vi "Estimate Signal Amplitude and Offset - Sine.vi"(9 "number of bits":i32, 10 "ideal code width":dbl, 11 "histogram":i32[](array[numeric])) -> (2 "estimated offset":dbl, 3 "estimated amplitude (pk-pk)":dbl)   [LabVIEW 2021]
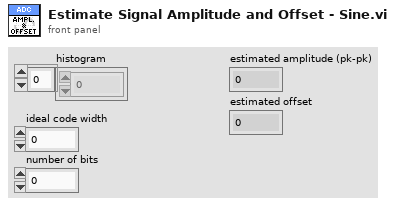
[diagram p1: front panel]
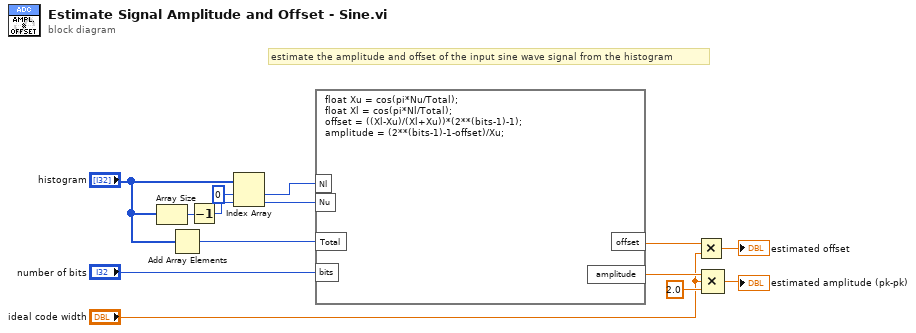
[diagram p0: block diagram]
diagram:
  # "estimate the amplitude and offset of the input sine wave signal from the histogram"
  n1 = Array Size(array="histogram") -> (size(s)=w14:i32)
  n2 = Add Array Elements(numeric array="histogram") -> (sum=w9:i32)
  n3 = Decrement(x=w14) -> (x-1=w13:i32)
  n4 = Index Array(array="histogram", index #1=0 ("index"), index #2=w13) -> (element #1=w11:i32, element #2=w10:i32)
  n5 = formula code="float Xu = cos(pi*Nu/Total);\nfloat Xl = cos(pi*Nl/Total);\noffset = ((Xl-Xu)/(Xl+Xu))*(2**(bits-1)-1);\namplitude = (2**(bits-1)-1-offset)/Xu;"("Nu"=w10, "Nl"=w11, "Total"=w9, "bits"="number of bits") -> ("offset"=w8:dbl, "amplitude"=w7:dbl)
  n6 = Multiply(x=w8, y="ideal code width") -> (x*y=→"estimated offset":dbl)
  n7 = Compound Arithmetic op=MULTIPLY(w7, "ideal code width", 2.0 ("value")) -> (→"estimated amplitude (pk-pk)":dbl)
